vi "Simple Add.vi"() -> ()   [LabVIEW 2017]
panel:
  out "Sum":dbl
  in  "z":dbl
  in  "y":dbl
  in  "x":dbl format="%#_13g"
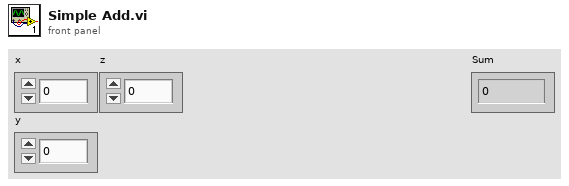
[diagram p1: front panel]
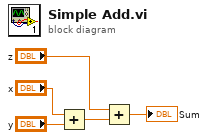
[diagram p0: block diagram]
diagram:
  n1 = Add(x="x", y="y") -> (x+y=w4:dbl)
  n2 = Add(x="z", y=w4) -> (x+y=→"Sum":dbl)
